vi "Subvi detector falling edge bool.vi"(10 "Input":bool) -> (2 "Output":bool)   [LabVIEW 2017]
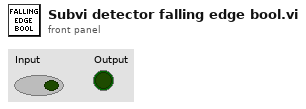
[diagram p1: front panel]
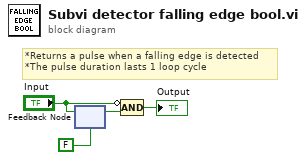
[diagram p0: block diagram]
diagram:
  # "*Returns a pulse when a falling edge is detected\n*The pulse duration lasts 1 loop cycle"
  n1 = feedback #1(FALSE ("Input")) -> (w3:bool)
  n2 = feedback-in #1("Input") -> ()
  n3 = Compound Arithmetic op=AND(invert "Input", w3) -> (→"Output":bool)
